vi "State.vi"(7 "Action":T2, 8 "Error In":errorcluster, 11 "Set Value":variant) -> (0 "Error Out":errorcluster, 3 "Data":T1)   [LabVIEW 2018, in "Toolkit.lvlib" / "Error.lvlib"]
uses:
  Error.lvlib
  Action.ctl
  Data.ctl
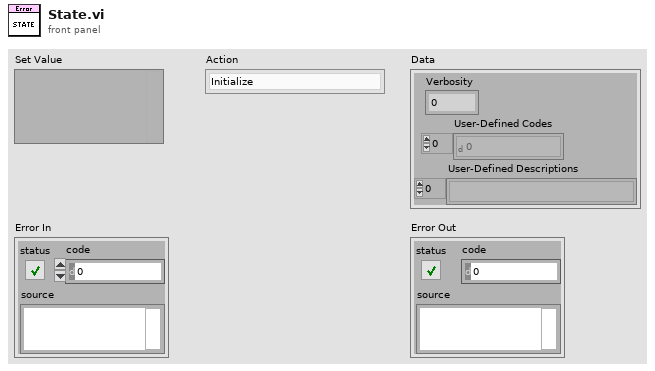
[diagram p1: front panel]
types:
  T1 = typedef "Toolkit.lvlib/Error.lvlib/Data.ctl" = cluster{"Verbosity":u8, "User-Defined Codes":i32[], "User-Defined Descriptions":string[]}
  T2 = typedef "Toolkit.lvlib/Error.lvlib/Action.ctl" = enum16{"Initialize", "Get", "Set Verbosity", "Set User-Defined Codes", "Set User-Defined Descriptions", "Shutdown"}
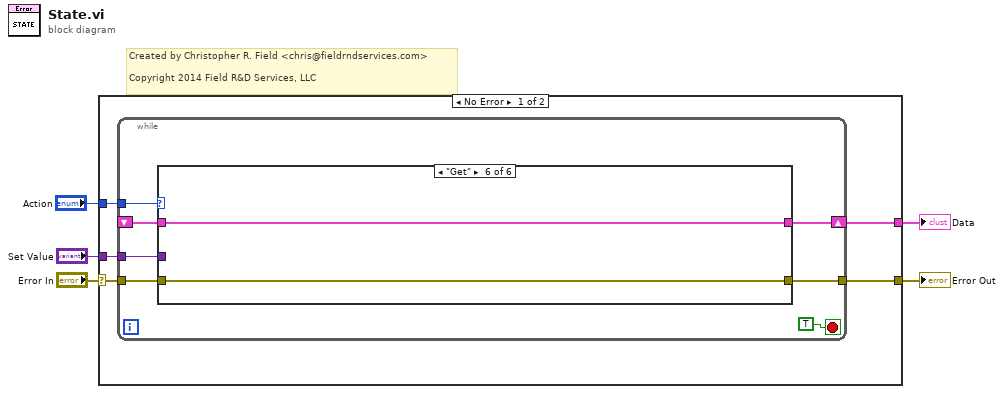
[diagram p0: block diagram]
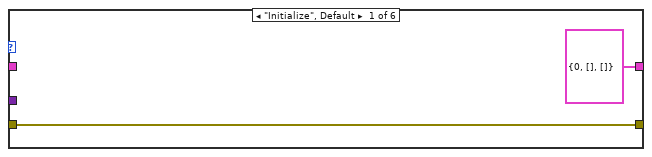
[diagram p2: hidden frame]
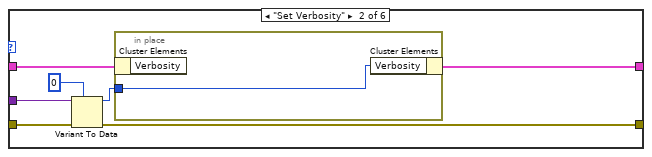
[diagram p3: hidden frame]
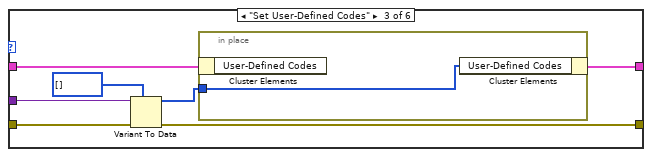
[diagram p4: hidden frame]
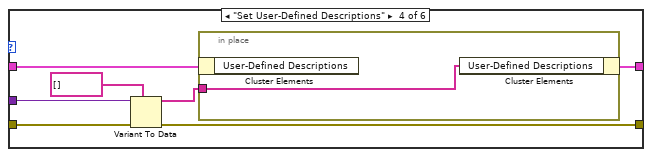
[diagram p5: hidden frame]
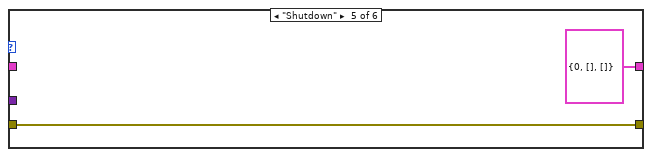
[diagram p6: hidden frame]
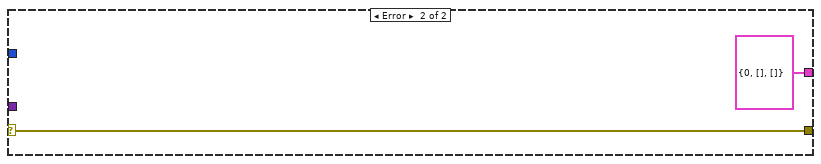
[diagram p7: hidden frame]
diagram:
  # "Created by Christopher R. Field <chris@fieldrndservices.com>\n\nCopyright 2014 Field R&D Services, LLC"
  n1 = case shown="No Error" "Error In" {
    selector: "Error In" -> [w9 w49]
    tunnel: "Action" -> [w10 _]
    tunnel: [w8 w49] -> w3
    tunnel: [w7 T1 {"Verbosity"=0, "User-Defined Codes"=[], "User-Defined Descriptions"=[]} ("Data")] -> w2
    tunnel: "Set Value" -> [w6 _]
    frame No Error {
      n2 = while {
        tunnel: w10 -> [w16]
        tunnel: w9 -> [w15]
        tunnel: [w14] -> w8
        shift-right: [w13] -> w7
        shift-left: _ -> [w12]
        tunnel: w6 -> [w11]
        stop <- TRUE stop-if-true
        n3 = case shown="\"Get\"" w16 {
          tunnel: w15 -> [w19 w25 w33 w41 w45 w47]
          tunnel: [w19 w24 w32 w40 w45 w47] -> w14
          tunnel: [T1 {"Verbosity"=0, "User-Defined Codes"=[], "User-Defined Descriptions"=[]} ("Data") w23 w31 w39 T1 {"Verbosity"=0, "User-Defined Codes"=[], "User-Defined Descriptions"=[]} ("Data") w46] -> w13
          tunnel: w12 -> [_ w26 w34 w42 _ w46]
          tunnel: w11 -> [_ w22 w30 w38 _ _]
          frame "Initialize", Default {
          }
          frame "Set Verbosity" {
            n4 = Variant To Data(error in=w25, type=u8 0 ("Verbosity"), Variant=w22) -> (data=w20:u8, error out=w24:errorcluster)
            n5 = in-place {
              in-place-border: w20 -> [w27]
              n6 = in-place-cluster #1(w26) -> ()  [unwired: 1 out]
              n7 = in-place-cluster #1("Verbosity"=w27) -> (w23:T1)
            }
          }
          frame "Set User-Defined Codes" {
            n8 = Variant To Data(error in=w33, type=i32[] [] ("User-Defined Codes"), Variant=w30) -> (data=w29:i32[], error out=w32:errorcluster)
            n9 = in-place {
              in-place-border: w29 -> [w35]
              n10 = in-place-cluster #2(w34) -> ()  [unwired: 1 out]
              n11 = in-place-cluster #2("User-Defined Codes"=w35) -> (w31:T1)
            }
          }
          frame "Set User-Defined Descriptions" {
            n12 = Variant To Data(error in=w41, type=string[] [] ("User-Defined Descriptions"), Variant=w38) -> (data=w37:string[], error out=w40:errorcluster)
            n13 = in-place {
              in-place-border: w37 -> [w43]
              n14 = in-place-cluster #3(w42) -> ()  [unwired: 1 out]
              n15 = in-place-cluster #3("User-Defined Descriptions"=w43) -> (w39:T1)
            }
          }
          frame "Shutdown" {
          }
          frame "Get" {
          }
        }
      }
    }
    frame Error {
    }
  }
  "Error Out" <- w3
  "Data" <- w2
